vi "PathPlanner_ConstraintsZone_ForSegmentIndex.vi"(9 "SegmentIndex":i32, 11 "ConstraintsZone":T1) -> (3 "new Constraints Zone":T1)   [LabVIEW 2019, in "PathPlanner24.lvlib"]
doc: "/**\n * Create a new path constraints object\n *\n * @param maxVelocityMps Max linear velocity (M/S)\n * @param maxAccelerationMpsSq Max linear acceleration (M/S^2)\n * @param maxAngularVelocityRps Max angular velocity (Rad/S)\n * @param maxAngularAccelerationRpsSq Max angular acceleration (Rad/S^2)\n */"
uses:
  PathPlanner24.lvlib
  TypeDef/PathPlannerConstraints.ctl
  TypeDef/PathPlannerConstraintsZone.ctl
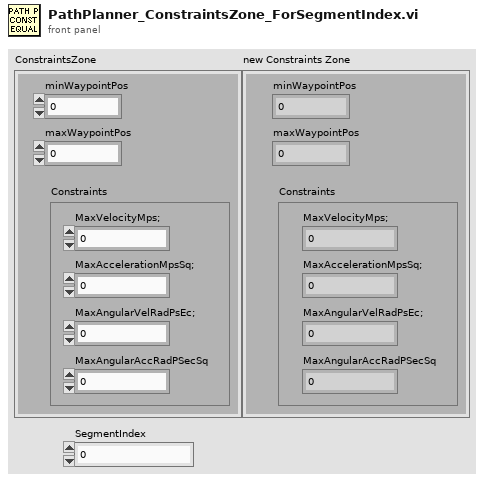
[diagram p1: front panel]
types:
  T1 = typedef "PathPlanner24.lvlib/PathPlannerConstraintsZone.ctl" = cluster{"minWaypointPos":dbl, "maxWaypointPos":dbl, "Constraints":T2}
  T2 = typedef "PathPlanner24.lvlib/PathPlannerConstraints.ctl" = cluster{"MaxVelocityMps;":dbl, "MaxAccelerationMpsSq;":dbl, "MaxAngularVelRadPsEc;":dbl, "MaxAngularAccRadPSecSq":dbl}
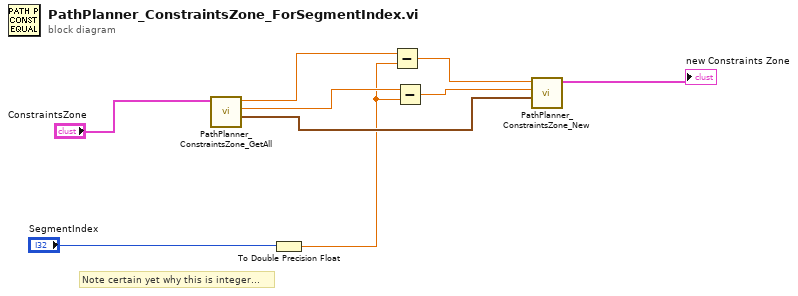
[diagram p0: block diagram]
diagram:
  # "Note certain yet why this is integer..."
  n1 = call "PathPlanner_ConstraintsZone_GetAll.vi"("ConstraintsZone"="ConstraintsZone") -> ("Constraints"=w6:T2, "maxWaypointPos"=w3:dbl, "minWaypointPos"=w7:dbl)  [unwired: 8 in]
  n2 = To Double Precision Float(number="SegmentIndex") -> (double precision float=w1:dbl)
  n3 = Subtract(x=w7, y=w1) -> (x-y=w5:dbl)
  n4 = Subtract(x=w3, y=w1) -> (x-y=w2:dbl)
  n5 = call "PathPlanner_ConstraintsZone_New.vi"("Constraints"=w6, "maxWaypointPos"=w2, "minWaypointPos"=w5) -> ("ConstraintsZone"=→"new Constraints Zone":T1)  [unwired: 8 in]
